vi "test_RemoteDigitalSession_CallCloseMeasurementLinkSessionWithDetachBehavior_RemoteSessionDetached.vi"(8 "error in":errorcluster) -> (0 "error out":errorcluster, 2 "result":string, 3 "pass":bool)   [LabVIEW 2020, in "MeasurementServerTests.lvlib"]
uses:
  MeasurementServerTests.lvlib
  Runtime/MeasurementLink Instrument/IInstrument/Close Session Behavior.ctl
  Runtime/MeasurementLink Instrument/IInstrument/IInstrument.lvclass
  Runtime/MeasurementLink niDigital/Instrument/Instrument.lvclass
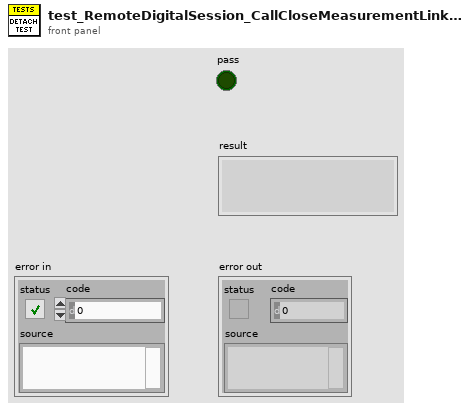
[diagram p1: front panel]
types:
  T1 = typedef "MeasurementLink Instrument.lvlib/IInstrument.lvclass/Remote Connection Options.ctl" = cluster{"session name":string, "address":string, "port":u32}
  T2 = typedef "MeasurementLink Instrument.lvlib/IInstrument.lvclass/Close Session Behavior.ctl" = enum16{"Close Session", "Detach Session"}
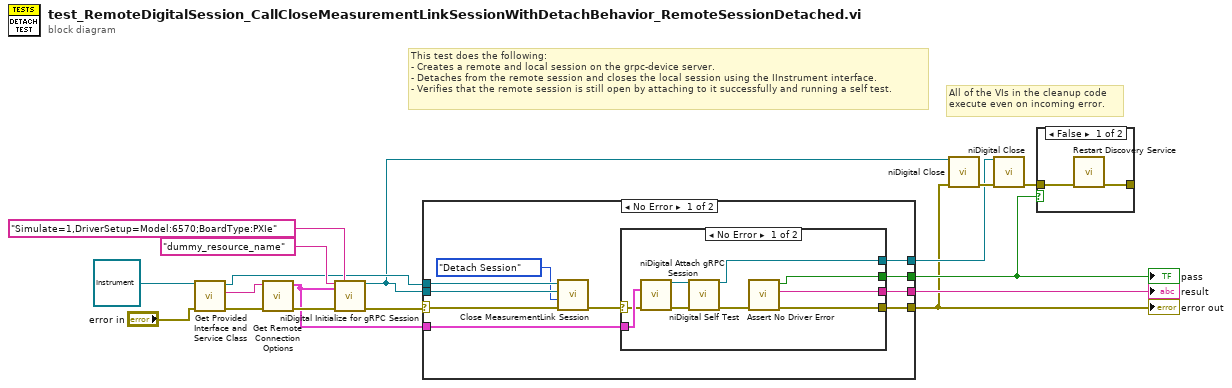
[diagram p0: block diagram]
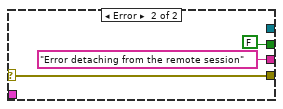
[diagram p2: hidden frame]
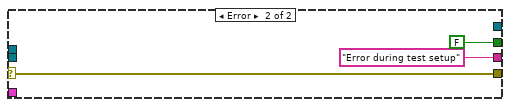
[diagram p3: hidden frame]
diagram:
  # "All of the VIs in the cleanup code\nexecute even on incoming error."
  # "This test does the following:\n- Creates a remote and local session on the grpc-device server.\n- Detaches from the remote session and closes the local session using the IInstrument interface.\n- Verifies that the remote session is still open by attaching to it successfully and running a self test."
  n1 = call-dynamic "Get Provided Interface and Service Class.vi"("error in"="error in", "instrument in"=refnum<class "Instrument.lvclass"> refnum ("MeasurementLink niDigital.lvlib:Instrument.lvclass")) -> ("error out"=w15:errorcluster, "provided interface"=w14:string, "instrument out"=w10:refnum<class "Instrument.lvclass">)  [unwired: 6 in, 1 out]
  n2 = call "Get Remote Connection Options.vi"("error in"=w15, "provided interface"=w14) -> ("error out"=w16:errorcluster, "remote connection options"=w9:T1)  [unwired: 8 in]
  n3 = call <instrlib>:"niDigital Initialize for gRPC Session.vi"("resource name"="dummy_resource_name", "option string"="Simulate=1,DriverSetup=Model:6570;BoardType:PXIe", "gRPC options"=w9, "error in"=w16) -> ("instrument handle"=w4:refnum<k15>, "error out"=w11:errorcluster)  [unwired: 10 in]
  n4 = case shown="No Error" w11 {
    selector: w11 -> [w27 w41]
    tunnel: w10 -> [w26 _]
    tunnel: w4 -> [w25 _]
    tunnel: w9 -> [w24 _]
    tunnel: [w22 w41] -> w2
    tunnel: [w21 FALSE] -> w5
    tunnel: [w20 "Error during test setup" ("f")] -> w8
    tunnel: [w18 _] -> w3
    frame No Error {
      n5 = call-dynamic "Close MeasurementLink Session.vi"("error in"=w27, "close session behavior"=Close_Session_Behavior."Detach Session", "session in"=w25, "instrument in"=w26) -> ("error out"=w23:errorcluster)  [unwired: 7 in]
      n6 = case shown="No Error" w23 {
        selector: w23 -> [w35 w37]
        tunnel: w24 -> [w36 _]
        tunnel: [w30 w37] -> w22
        tunnel: [w28 FALSE] -> w21
        tunnel: [w29 "Error detaching from the remote session" ("f")] -> w20
        tunnel: [w32 _] -> w18
        frame No Error {
          n7 = call <instrlib>:"niDigital Attach gRPC Session.vi"("gRPC options"=w36, "error in"=w35) -> ("instrument handle out"=w34:refnum<k15>, "error out"=w33:errorcluster)  [unwired: 12 in]
          n8 = call <instrlib>:"niDigital Self Test.vi"("instrument handle in"=w34, "error in"=w33) -> ("instrument handle out"=w32:refnum<k15>, "error out"=w31:errorcluster)  [unwired: 10 in, 2 out]
          n9 = call "Assert No Driver Error.vi"("error in"=w31) -> ("error out"=w30:errorcluster, "result"=w29:string, "pass?"=w28:bool)  [unwired: 8 in]
        }
        frame Error {
        }
      }
    }
    frame Error {
    }
  }
  "error out" <- w2
  "pass" <- w5
  "result" <- w8
  n10 = call <instrlib>:"niDigital Close.vi"("instrument handle"=w4, "error in"=w2) -> ("error out"=w7:errorcluster)  [unwired: 13 in]
  n11 = call <instrlib>:"niDigital Close.vi"("instrument handle"=w3, "error in"=w7) -> ("error out"=w6:errorcluster)  [unwired: 13 in]
  n12 = case shown="False" w5 {
    tunnel: [w44 _] -> _
    tunnel: w6 -> [w43 _]
    frame False {
      n13 = call "Restart Discovery Service.vi"("error in"=w43) -> ("error out"=w44:errorcluster)  [unwired: 10 in]
    }
    frame True {
    }
  }
